vi "Calculate ROI component's time.vi"(9 "AOD fill time (us)":dbl=24.4, 11 "Normalised ROI setup":T1 {"ROI group ID" format="%#_6f"; "Laser Power (%)" format="%#_6f"; "Zoom" format="%#_6f"; "Frame Size" format="%#_6f"; "Number of lines" format="%#_6f"; "Composite ID" format="%#_6f"; "Angle (deg)" format="%#_6f"; "ROI Time (ns)" format="%#_6f"; "ROI ID" format="%#_6f"; "Pixels in ROI" format="%#_6f"; "ROI index" format="%#_6f"; "Z stop" format="%#_6f"; "Y stop" format="%#_6f"; "X stop" format="%#_6f"; "Z start" format="%#_6f"; "X start" format="%#_6f"; "Y start" format="%#_6f"}) -> (3 "ROI component's time (us)":dbl)   [LabVIEW 2013]
uses:
  User Interface/Visualisation/Functional Imaging Viewer/Typedefs/ROI parameters data type.ctl
  Typedefs/ROI ID Enum.ctl
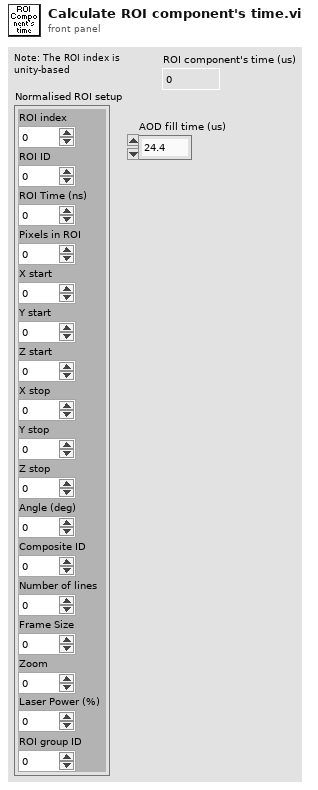
[diagram p1: front panel]
types:
  T1 = typedef "ROI parameters data type.ctl" = cluster{"ROI index":dbl, "ROI ID":dbl, "ROI Time (ns)":dbl, "Pixels in ROI":dbl, "X start":dbl, "Y start":dbl, "Z start":dbl, "X stop":dbl, "Y stop":dbl, "Z stop":dbl, "Angle (deg)":dbl, "Composite ID":dbl, "Number of lines":dbl, "Frame Size":dbl, "Zoom":dbl, "Laser Power (%)":dbl, "ROI group ID":dbl}
  T2 = typedef "ROI ID Enum.ctl" = enum16{"Point", "MiniScan", "Comp. MiniScan", "Rectangle", "Comp. volume", "Arb. plane point"}
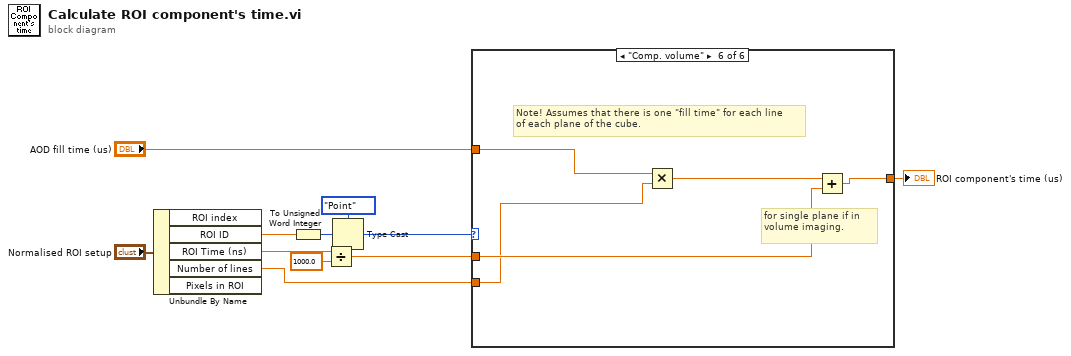
[diagram p0: block diagram]
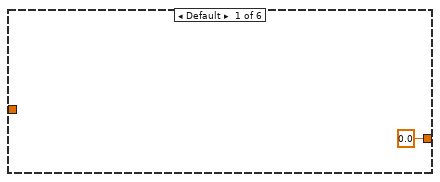
[diagram p2: hidden frame]
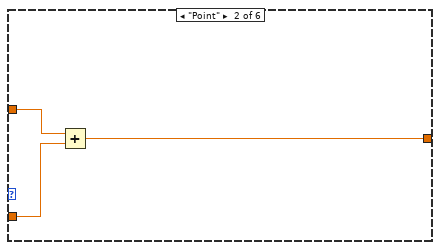
[diagram p3: hidden frame]
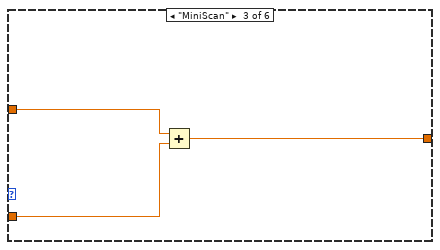
[diagram p4: hidden frame]
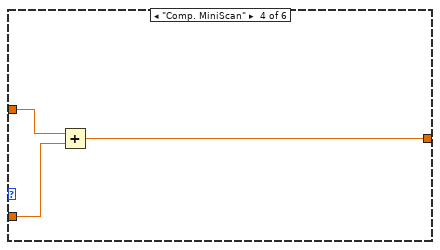
[diagram p5: hidden frame]
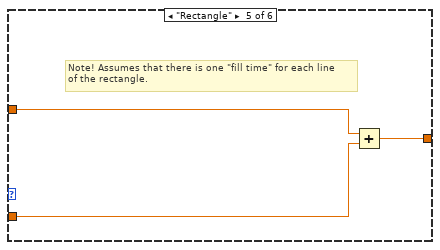
[diagram p6: hidden frame]
diagram:
  n1 = Unbundle By Name("Normalised ROI setup") -> ("ROI ID"=w2:dbl, "ROI Time (ns)"=w7:dbl, "Number of lines"=w9:dbl)  [unwired: 2 out]
  n2 = To Unsigned Word Integer(number=w2) -> (unsigned 16bit integer=w4:u16)
  n3 = Divide(x=w7, y=1000.0) -> (x/y=w8:dbl)
  n4 = Type Cast(type=ROI_ID_Enum."Point" ("ROI ID Enum"), x=w4) -> (*(type *) &x=w5:T2)
  n5 = case shown="\"Comp. volume\"" w5 {
    tunnel: w8 -> [_ w15 w18 w21 w24 w29]
    tunnel: "AOD fill time (us)" -> [_ w14 w17 w20 w23 w28]
    tunnel: [0.0 w13 w16 w19 w22 w25] -> w10
    tunnel: w9 -> [_ _ _ _ _ w27]
    frame Default {
    }
    frame "Point" {
      n6 = Add(x=w14, y=w15) -> (x+y=w13:dbl)
    }
    frame "MiniScan" {
      n7 = Add(x=w17, y=w18) -> (x+y=w16:dbl)
    }
    frame "Comp. MiniScan" {
      n8 = Add(x=w20, y=w21) -> (x+y=w19:dbl)
    }
    frame "Rectangle" {
      # "Note! Assumes that there is one \"fill time\" for each line\nof the rectangle."
      n9 = Add(x=w23, y=w24) -> (x+y=w22:dbl)
    }
    frame "Comp. volume" {
      # "for single plane if in volume imaging."
      # "Note! Assumes that there is one \"fill time\" for each line\nof each plane of the cube."
      n10 = Multiply(x=w28, y=w27) -> (x*y=w26:dbl)
      n11 = Add(x=w26, y=w29) -> (x+y=w25:dbl)
    }
  }
  "ROI component's time (us)" <- w10
